vi "stepperTest.vi"() -> ()   [LabVIEW 2019]
uses:
  <vilib>/Platform/TimedLoop/XDataNode/timing_clust.ctl
  <vilib>/Platform/TimedLoop/XDataNode/nitl_modes.ctl
  <vilib>/Platform/TimedLoop/XDataNode/wakeup.ctl
  <vilib>/platform/TimedLoop/XDataNode/XDataNode.xnode
  <vilib>/Platform/TimedLoop/XDataNode/XDNodeRunTimeDep.lvlib
panel:
  in  "Speed (deg/s)":dbl(slide) scale=-1000.0..1000.0
  in  "Sine?":bool
  out "error out (no error) 2":errorcluster
  out "error out (no error)":errorcluster
  in  "Stop Button":bool
  out "Waveform Chart":dbl(graph)
  in  "y 2":dbl
  in  "y":dbl
  out "DegreeCounter":dbl
  in  "EN [L,R]":bool
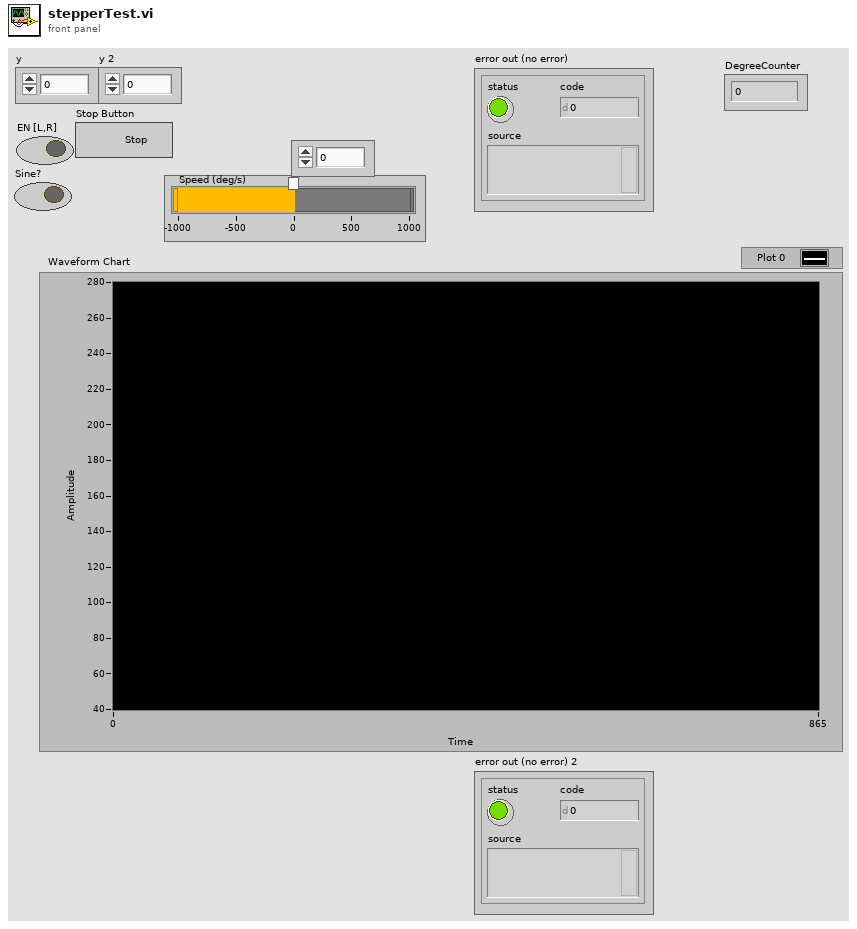
[diagram p1: front panel]
types:
  T1 = typedef "miniRef.ctl" = cluster{"Custom FPGA Reference":refnum<k20>, "error out":errorcluster}
  T2 = typedef "XDNodeRunTimeDep.lvlib/timing_clust.ctl" = cluster{"Expected End [f-1]":u64, "Actual End [f-1]":u64, "Finished Late? [f-1]":bool, "Expected End [i-1]":u64, "Actual End [i-1]":u64, "Finished Late? [i-1]":bool, "Expected Start [i]":u64, "Actual Start [i]":u64, "Expected Start [f]":u64, "Actual Start [f]":u64, "Source Name":string, "Structure Name":string, "Period":i64, "Deadline":i64, "Offset":i64, "Start":i64, "Priority":i32, "Timeout":i32, "Mode":T3, "Wakeup Reason":T4, "Error":errorcluster, "Source Type":string, "Secondary Source Type":string, "Global End Time":u64, "Global Start Time":u64, "Frame Duration":u64, "Iteration Duration":u64, "Assigned CPU":i32, "I/O Scan Engine Mode":u32}
  T3 = typedef "XDNodeRunTimeDep.lvlib/nitl_modes.ctl" = enum32{"No Change", "Process missed periods, maintain original phase", "Discard missed periods, maintain original phase", "Process missed periods, ignore original phase", "Discard missed periods, ignore original phase"}
  T4 = typedef "XDNodeRunTimeDep.lvlib/wakeup.ctl" = enum32{"Normal", "Aborted", "Asynchronous wakeup", "Timing source error", "Timed loop error", "Timeout"}
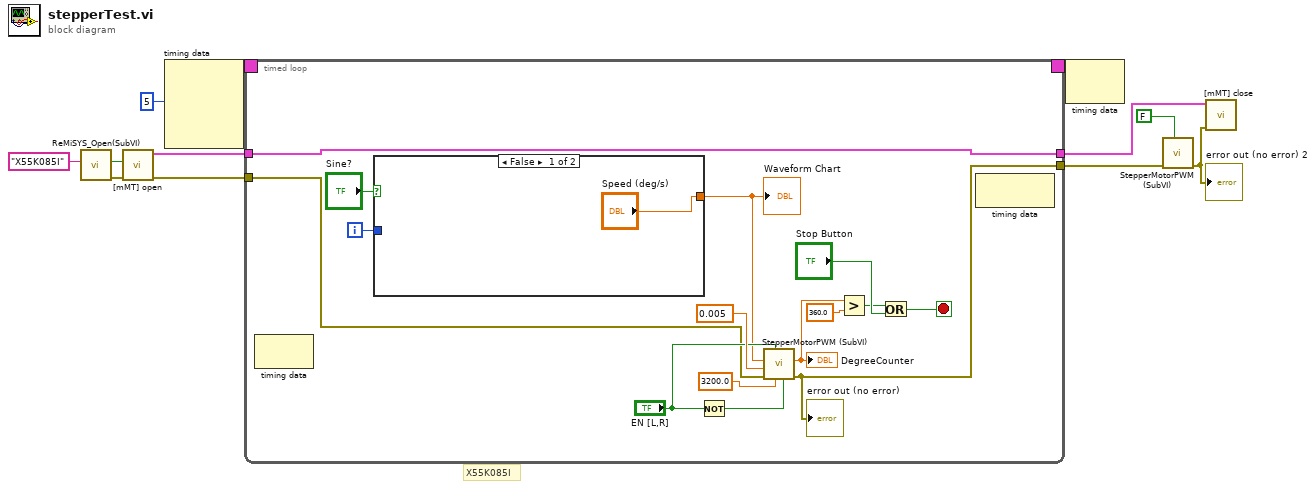
[diagram p0: block diagram]
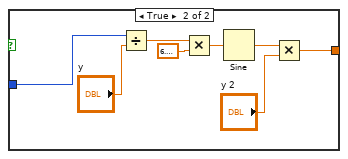
[diagram p2: hidden frame]
diagram:
  # "X55K085I"
  n1 = call <vilib>:"ReMiSYS_Open(SubVI).vi"("ReMiSYS Key"="X55K085I") -> ("error out"=w7:errorcluster, "Correct Key?"=w6:bool)  [unwired: 9 in]
  n2 = call <vilib>:"[mMT] open.vi"("error in"=w7, "Servo6,7"=w6) -> ("error out"=w5:errorcluster, "miniOut"=w3:T1)  [unwired: 7 in, 1 out]
  n3 = node-c288(i64 5 ("Period")) -> (w12:T2)  [unwired: 3 in]
  n4 = timed-loop {
    timing: w12 -> [_]
    timing-out: [_] -> w11
    tunnel: [w27] -> w9
    tunnel: w5 -> [w14]
    tunnel: [w15] -> w4
    tunnel: w3 -> [w15]
    i -> [w21]
    stop <- w17 stop-if-true
    n5 = node-c288() -> ()  [unwired: 1 in, 1 out]
    n6 = case shown="False" "Sine?" {
      tunnel: w21 -> [_ w36]
      tunnel: ["Speed (deg/s)" w31] -> w20
      frame False {
      }
      frame True {
        n7 = Divide(x=w36, y="y") -> (x/y=w35:dbl)
        n8 = Multiply(x=w35, y=6.283185307179586) -> (x*y=w34:dbl)
        n9 = Sine(x=w34) -> (sin(x)=w32:dbl)
        n10 = Multiply(x=w32, y="y 2") -> (x*y=w31:dbl)
      }
    }
    "Waveform Chart" <- w20
    n11 = Not(x="EN [L,R]") -> (.not. x?=w24:bool)
    n12 = call "StepperMotorPWM (SubVI).vi"("Reset"=w24, "steps/rev"=3200.0, "EN"="EN [L,R]", "error in (no error)"=w14, "LoopTime"=0.005, "Speed (deg/s) [L,R]"=w20) -> ("error out (no error)"=w27:errorcluster, "DegreeCounter"=w23:dbl)  [unwired: 4 in]
    "DegreeCounter" <- w23
    "error out (no error)" <- w27
    n13 = Greater?(x=w23, y=360.0) -> (0:w18:bool)
    n14 = Or(x=w18, y="Stop Button") -> (x .or. y?=w17:bool)
    n15 = node-c288() -> ()  [unwired: 1 in, 1 out]
  }
  n16 = node-c288(w11) -> ()  [unwired: 1 out]
  n17 = call "StepperMotorPWM (SubVI).vi"("EN"=FALSE ("EN [L,R]"), "error in (no error)"=w9) -> ("error out (no error)"=w1:errorcluster)  [unwired: 8 in, 1 out]
  "error out (no error) 2" <- w1
  n18 = call <vilib>:"[mMT] close.vi"("error in (no error)"=w1, "miniOut in"=w4) -> ()  [unwired: 9 in, 1 out]
